vi "用鼠标选取曲线.vi"() -> ()   [LabVIEW 2011]
panel:
  in  "Stop Button":bool
  out "Waveform Graph":dbl[][](graph)
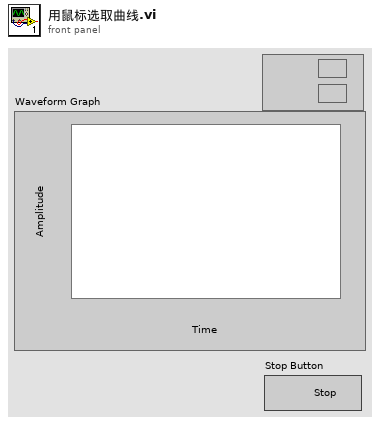
[diagram p1: front panel]
types:
  T1 = typedef "LVPoint32TypeDef.ctl" = cluster{"Horizontal":i32, "Vertical":i32}
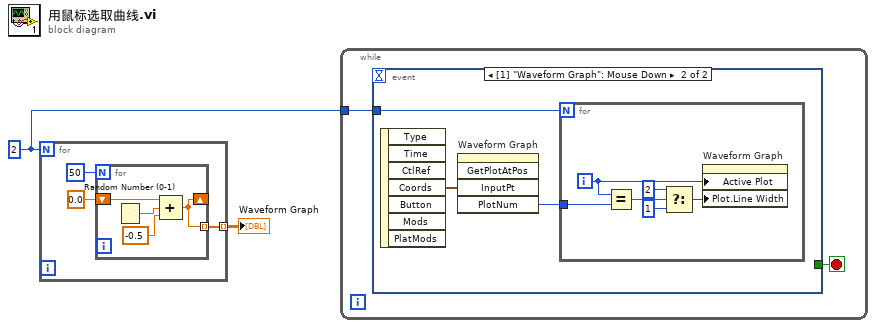
[diagram p0: block diagram]
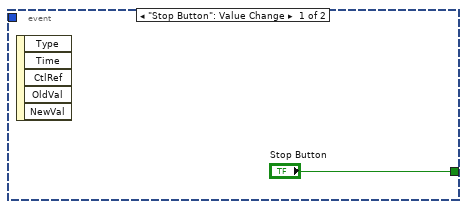
[diagram p2: hidden frame]
diagram:
  w1 = 2
  n1 = for {
    N: w1 -> [_]
    tunnel: [w3] -> w2 mode=indexing
    n2 = for {
      N: 50 -> [_]
      shift-right: [w7] -> _
      shift-left: 0.0 -> [w9]
      tunnel: [w7] -> w3 mode=indexing
      n3 = Random Number (0-1)() -> (number: 0 to 1=w8:dbl)
      n4 = Compound Arithmetic op=ADD(w9, w8, -0.5 ("value")) -> (w7:dbl)
    }
  }
  "Waveform Graph" <- w2
  n5 = while {
    tunnel: w1 -> [w10]
    stop <- w11 stop-if-true
    n6 = event shown="[1] \"Waveform Graph\": Mouse Down" {
      selector: _ -> [_ _]
      dyn-events: _ -> [_ _]
      timeout: _ -> [_ _]
      tunnel: ["Stop Button" _] -> w11
      tunnel: w10 -> [_ w14]
      event "Stop Button": Value Change {
        n7 = event-data() -> ()  [unwired: 1 in, 5 out]
      }
      event "Waveform Graph": Mouse Down {
        n8 = event-data() -> ("Coords"=w15:T1)  [unwired: 1 in, 6 out]
        n9 = invoke on="Waveform Graph" class="WFGraph (strict)" method="GetPlotAtPos"("InputPt"=w15) -> ("PlotNum"=w13:i32)  [unwired: 4 in, 4 out]
        n10 = for {
          N: w14 -> [_]
          tunnel: w13 -> [w21]
          i -> [w20]
          n11 = Equal?(x=w20, y=w21) -> (x = y?=w19:bool)
          n12 = Select(t=u8 2 ("Plot.Line Width"), s=w19, f=u8 1 ("Plot.Line Width")) -> (s? t:f=w16:u8)
          n13 = property on="Waveform Graph" class="WFGraph (strict)"("Active Plot"=w20, "Plot.Line Width"=w16) -> ()  [unwired: 2 in, 2 out]
        }
      }
    }
  }
